vi "Different Types.vi"() -> ()   [LabVIEW 2017, in "Assertions.Tests.lvlib" / "Assert In Range.lvlib"]
uses:
  Assert In Range.lvlib
  src/Transparent Assertions/Constraints/Logical And/Logical And.lvclass
  C:/Users/pasca/Projects/Home/TransparentAssertions/src/Transparent Assertions/Constraints/Binary Operator/Binary Operator.lvclass
  src/Transparent Assertions/Constraints/Logical Or/Logical Or.lvclass
  C:/Users/pasca/Projects/Home/TransparentAssertions/src/Transparent Assertions/Constraints/Constraint/Constraint.lvclass
  src/Transparent Assertions/Constraints/Is Less Than/Is Less Than.lvclass
  src/Transparent Assertions/Constraints/IsEqual/IsEqual.lvclass
  src/Transparent Assertions/Constraints/Is Greater Than/Is Greater Than.lvclass
  src/Transparent Assertions/Constraints/IsEqual/Create.vi
  src/Transparent Assertions/Constraints/Is Less Than/Create.vi
  src/Transparent Assertions/Constraints/Binary Operator/Create.vi
  src/Transparent Assertions/Constraints/Is Greater Than/Create.vi
  src/Transparent Assertions/Assertions/Assertions.lvlib
panel:
  out "error out":errorcluster
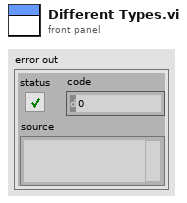
[diagram p1: front panel]
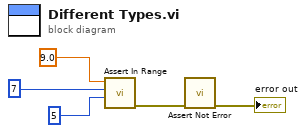
[diagram p0: block diagram]
diagram:
  n1 = call "Assert In Range.vi"("Minimum"=u16 5, "Actual"=7, "Maximum"=9.0) -> ("error out"=w2:errorcluster)  [unwired: 8 in]
  n2 = call "Assert Not Error.vi"("error in (no error)"=w2) -> ("error out"=→"error out":errorcluster)  [unwired: 10 in]
